vi "Signal synchronization v2.vi"() -> ()   [LabVIEW 2020]
uses:
  <vilib>/DAQmx/write.llb/DAQmx Write (Analog 1D Wfm NChan NSamp).vi
  <vilib>/DAQmx/create/channels.llb/DAQmx Create Channel (AO-Voltage-Basic).vi
  <vilib>/Analysis/1siggen.llb/Ramp Pattern by Delta.vi
  <vilib>/DAQmx/create/channels.llb/DAQmx Create Channel (CO-Pulse Generation-Frequency).vi
  <vilib>/DAQmx/configure/timing.llb/DAQmx Timing (Implicit).vi
  <vilib>/DAQmx/configure/timing.llb/DAQmx Timing (Use Waveform).vi
  <vilib>/DAQmx/miscellaneous.llb/DAQmx Fill In Error Info.vi
  <vilib>/Analysis/NI_AALBase.lvlib
panel:
  out "size(s) 2":i32
  out "size(s)":i32
  out "samples":i32
  out "x*y":dbl
  out "x/y":dbl
  out "Waveform Graph 4":waveform(dbl)[](graph)
  out "Waveform Graph 3":dbl[](graph)
  out "Waveform Graph 2":dbl[](graph)
  out "Waveform Graph":dbl[](graph)
  out "Ramp Array Size Final":i32
  out "Number of slices":dbl
  in  "End position (mm)":dbl
  out "Total Z thickness (mm)":dbl
  in  "Z slice width (mm)":dbl
  in  "Start position(mm)":dbl
  out "number of samples written per channel":u32
  in  "stop":bool
  # "Fs = sampling rate (samples/sec)\n#s= number of samples in the waveform"
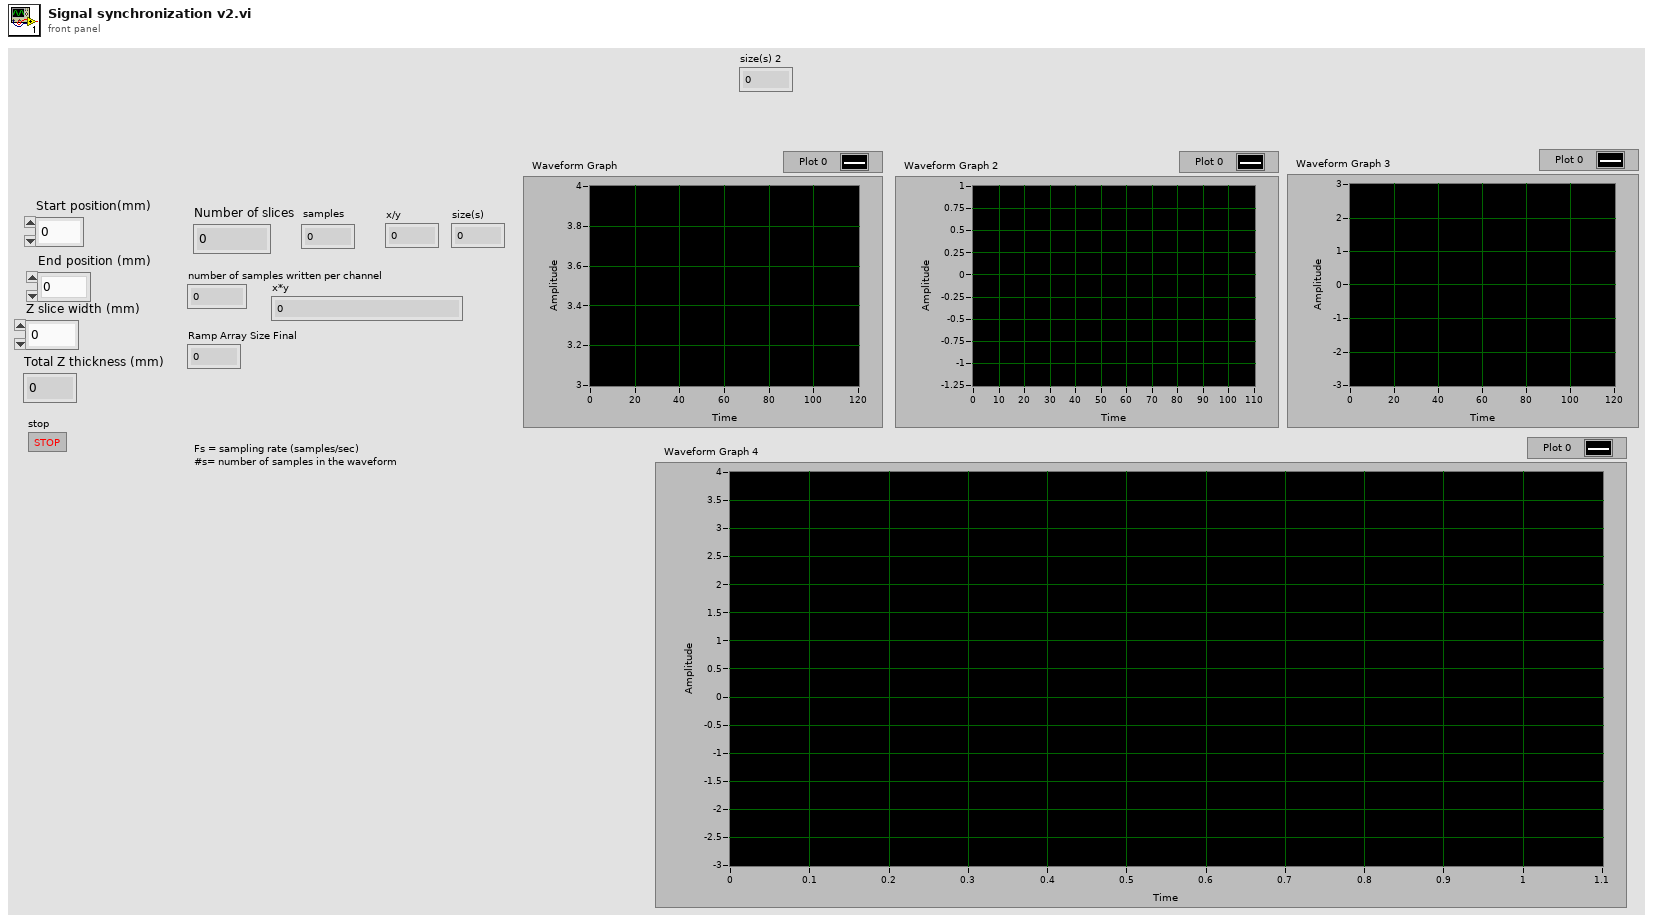
[diagram p1: front panel]
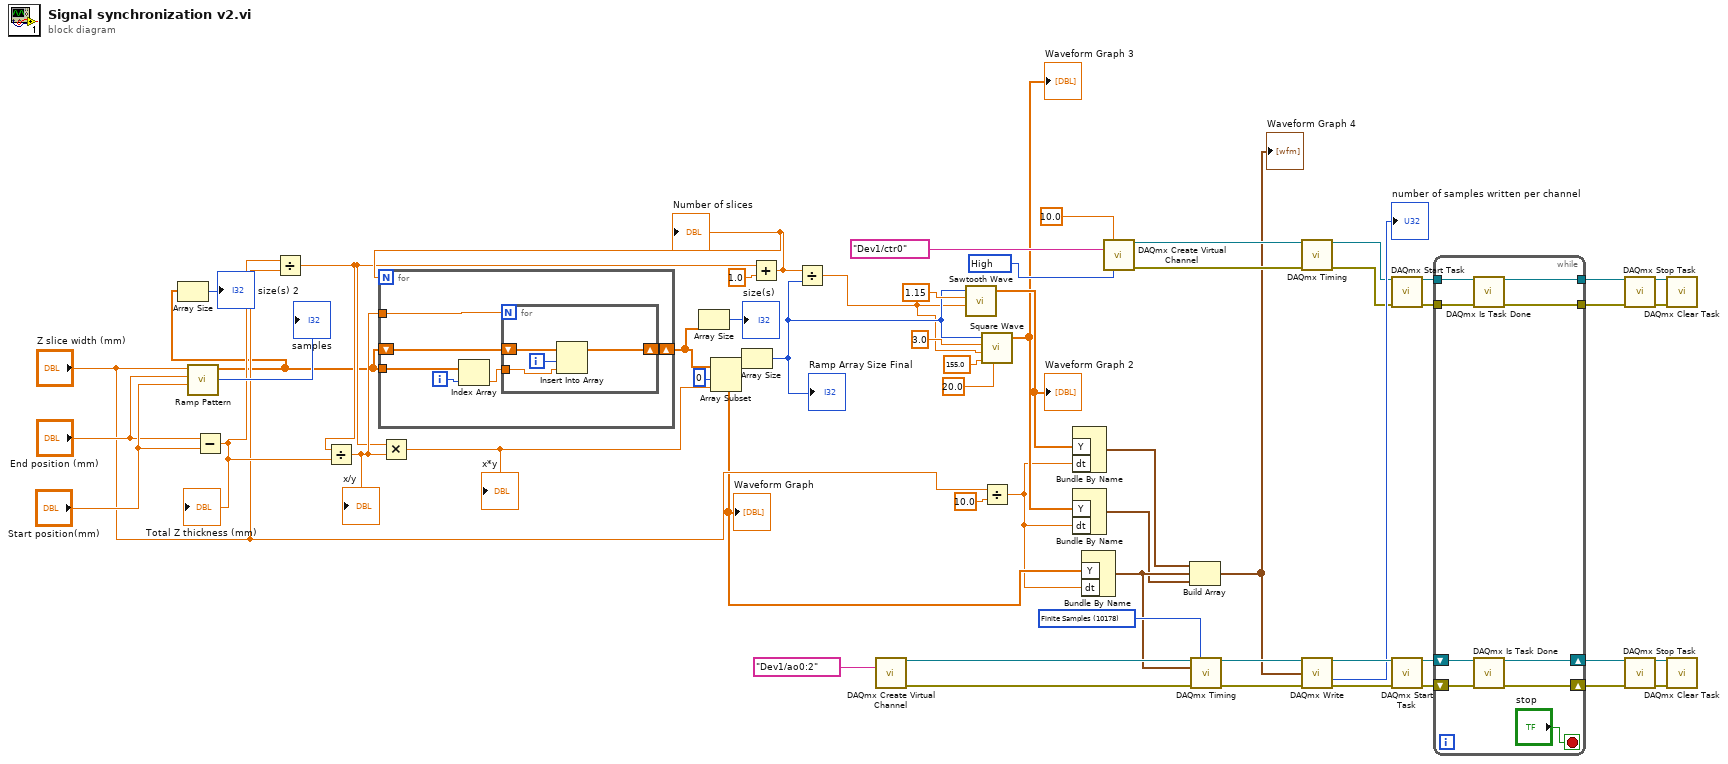
[diagram p0: block diagram]
diagram:
  w26 = 10192 items=["High"=10192, "Low"=10214] ("idle state")
  w51 = 10178 items=["Finite Samples"=10178, "Continuous Samples"=10123, "Hardware Timed Single Point"=12522] ("sample mode")
  n1 = call-poly <vilib>:"Ramp Pattern.vi"("start"="Start position(mm)", "end"="End position (mm)", "delta"="Z slice width (mm)") -> ("samples"=→"samples":i32, "Ramp Pattern"=w2:dbl[])  [unwired: 6 in, 1 out]
  n2 = Array Size(array=w2) -> (size(s)=→"size(s) 2":i32)
  n3 = Subtract(x="End position (mm)", y="Start position(mm)") -> (x-y=w21:dbl)
  "Total Z thickness (mm)" <- w21
  n4 = Divide(x=w21, y="Z slice width (mm)") -> (x/y=w5:dbl)
  n5 = Divide(x=w5, y=w21) -> (x/y=w23:dbl)
  "x/y" <- w23
  n6 = Multiply(x=w5, y=w23) -> (x*y=w38:dbl)
  "x*y" <- w38
  n7 = Add(x=w5, y=1.0) -> (x+y=w7:dbl)
  "Number of slices" <- w7
  n8 = for {
    N: w7 -> [_]
    shift-right: [w64] -> w4
    shift-left: w2 -> [w63]
    tunnel: w2 -> [w62]
    tunnel: w23 -> [w59]
    i -> [w60]
    n9 = Index Array "Index Array"(array=w62, index=w60) -> (element=w61:dbl)
    n10 = for {
      N: w59 -> [_]
      shift-right: [w67] -> w64
      shift-left: w63 -> [w68]
      tunnel: w61 -> [w65]
      i -> [w66]
      n11 = Insert Into Array "Insert Into Array"(array=w68, index=w66, new element=w65) -> (w67:dbl[])
    }
  }
  n12 = Array Size(array=w4) -> (size(s)=→"size(s)":i32)
  n13 = Array Subset(array=w4, index=0, length=w38) -> (w10:dbl[])
  "Waveform Graph" <- w10
  n14 = Array Size(array=w10) -> (size(s)=w16:i32)
  "Ramp Array Size Final" <- w16
  n15 = Divide(x=w7, y=w16) -> (x/y=w6:dbl)
  n16 = call-poly <vilib>:"DAQmx Create Virtual Channel.vi"("physical channels"=tag "Dev1/ao0:2") -> ("task out"=w58:refnum<k21>, "error out"=w57:errorcluster)  [unwired: 13 in]
  n17 = call <vilib>:"Sawtooth Wave.vi"("samples"=w16, "amplitude"=1.15, "frequency"=w6) -> ("sawtooth wave"=w13:dbl[])  [unwired: 2 in, 2 out]
  "Waveform Graph 2" <- w13
  n18 = call <vilib>:"Square Wave.vi"("samples"=w16, "amplitude"=3.0, "frequency"=w6, "duty cycle (%)"=20.0, "phase in"=155.0) -> ("square wave"=w12:dbl[])  [unwired: 1 in, 2 out]
  "Waveform Graph 3" <- w12
  n19 = Divide(x="Z slice width (mm)", y=10.0) -> (x/y=w8:dbl)
  n20 = Bundle By Name("Y"=w13, "dt"=w8) -> (w22:waveform(dbl))  [unwired: 1 in]
  n21 = Bundle By Name("Y"=w12, "dt"=w8) -> (w14:waveform(dbl))  [unwired: 1 in]
  n22 = Bundle By Name("Y"=w10, "dt"=w8) -> (w45:waveform(dbl))  [unwired: 1 in]
  n23 = call-poly <vilib>:"DAQmx Create Virtual Channel.vi"("frequency"=10.0, "counter"=tag "Dev1/ctr0", "idle state"=w26) -> ("task out"=w36:refnum<k21>, "error out"=w35:errorcluster)  [unwired: 11 in]
  n24 = Build Array(w22, w45, w14) -> (w11:waveform(dbl)[])
  "Waveform Graph 4" <- w11
  n25 = call-poly <vilib>:"DAQmx Timing.vi"("task/channels in"=w58, "sample mode"=w51, "waveform"=w45, "error in"=w57) -> ("task out"=w49:refnum<k21>, "error out"=w46:errorcluster)  [unwired: 10 in]
  n26 = call-poly <vilib>:"DAQmx Timing.vi"("task/channels in"=w36, "error in"=w35) -> ("task out"=w34:refnum<k21>, "error out"=w33:errorcluster)  [unwired: 12 in]
  n27 = call-poly <vilib>:"DAQmx Write.vi"("task/channels in"=w49, "data"=w11, "error in"=w46) -> ("task out"=w44:refnum<k21>, "number of samples written per channel"=→"number of samples written per channel":u32, "error out"=w43:errorcluster)  [unwired: 10 in]
  n28 = call <vilib>:"DAQmx Start Task.vi"("task/channels in"=w34, "error in"=w33) -> ("task out"=w32:refnum<k21>, "error out"=w31:errorcluster)  [unwired: 12 in]
  n29 = call <vilib>:"DAQmx Start Task.vi"("task/channels in"=w44, "error in"=w43) -> ("task out"=w42:refnum<k21>, "error out"=w41:errorcluster)  [unwired: 12 in]
  n30 = while {
    shift-right: [w75] -> w55
    shift-left: w42 -> [w77]
    shift-right: [w74] -> w54
    shift-left: w41 -> [w76]
    tunnel: w32 -> [w72]
    tunnel: w31 -> [w71]
    tunnel: [w70] -> w28
    tunnel: [w69] -> w27
    stop <- "stop" stop-if-true
    n31 = call <vilib>:"DAQmx Is Task Done.vi"("task/channels in"=w72, "error in"=w71) -> ("task out"=w70:refnum<k21>, "error out"=w69:errorcluster)  [unwired: 11 in, 1 out]
    n32 = call <vilib>:"DAQmx Is Task Done.vi"("task/channels in"=w77, "error in"=w76) -> ("task out"=w75:refnum<k21>, "error out"=w74:errorcluster)  [unwired: 11 in, 1 out]
  }
  n33 = call <vilib>:"DAQmx Stop Task.vi"("task/channels in"=w28, "error in"=w27) -> ("task out"=w30:refnum<k21>, "error out"=w29:errorcluster)  [unwired: 12 in]
  n34 = call <vilib>:"DAQmx Stop Task.vi"("task/channels in"=w55, "error in"=w54) -> ("task out"=w53:refnum<k21>, "error out"=w52:errorcluster)  [unwired: 12 in]
  n35 = call <vilib>:"DAQmx Clear Task.vi"("task in"=w30, "error in"=w29) -> ()  [unwired: 13 in, 1 out]
  n36 = call <vilib>:"DAQmx Clear Task.vi"("task in"=w53, "error in"=w52) -> ()  [unwired: 13 in, 1 out]
